vi "initialize.vi"(0 "mode":i32) -> ()   [LabVIEW 2015]
uses:
  phlib.dll
panel:
  out "Serial[8]":string="**********"
  in  "String2[8]":string="**********"
  out "Returncode PH_Initialize":i32
  out "Returncode PH_GetHardwareVersion":i32
  in  "String3[16]":string="*****************"
  in  "String4[8]":string="**********"
  out "DLL Version":string
  in  "String1[8]":string="**********"
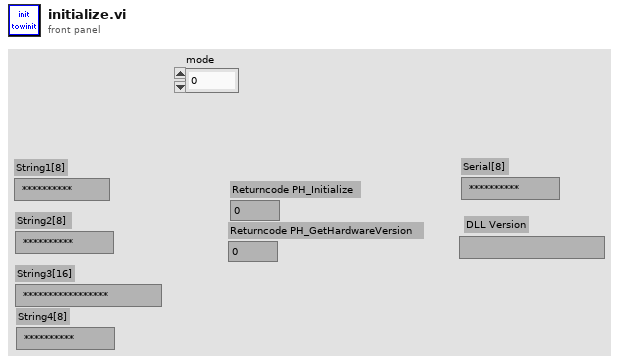
[diagram p1: front panel]
types:
  T1 = cluster{"initialized":bool, "devidx":i32, "Ch0 Level":i32, "Ch0 ZeroX":i32, "Ch1 Level":i32, "Ch1 ZeroX":i32, "sync rate":i32, "resolution":i32, "acq time":i32, "acq rate":i32, "# bins":u32, "Bin size":enum16{"1", "2", "4", "8", "16", "32", "64", "128"}, "min photons":u32, "truncate":u32}
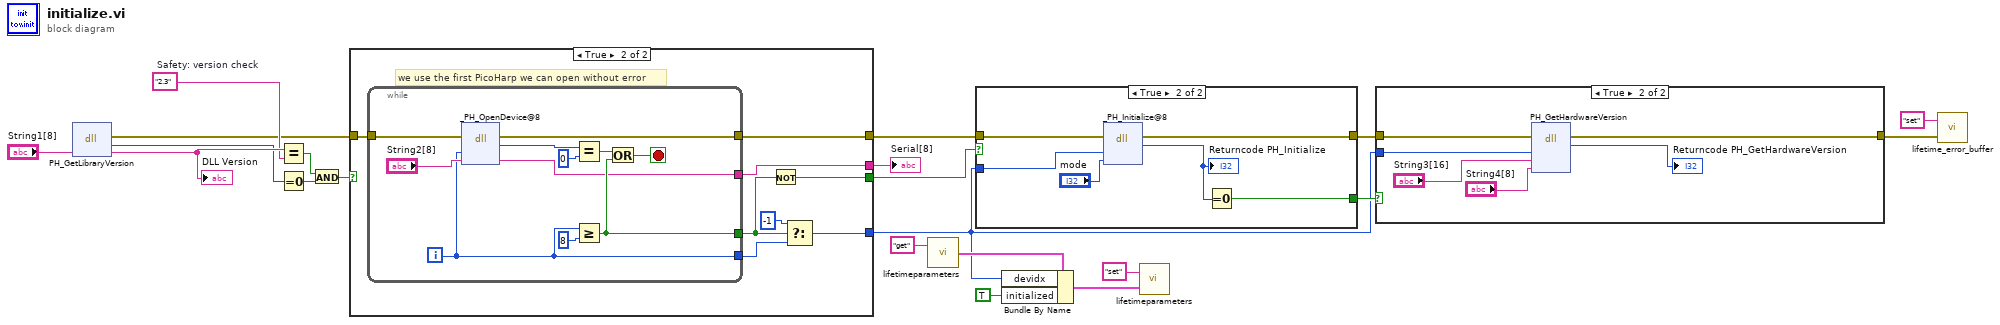
[diagram p0: block diagram]
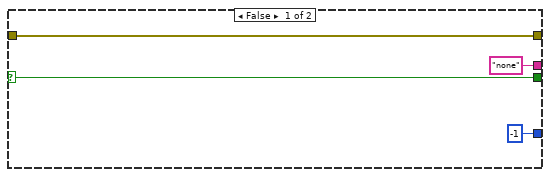
[diagram p2: hidden frame]
diagram:
  w19 = "2.3"  # Safety: version check
  n1 = dll-call lib="phlib.dll" fn="PH_GetLibraryVersion"("Version"="String1[8]") -> (error out=w5:errorcluster, w16:i32, "Version"=w20:string)  [unwired: 3 in, 1 out]
  "DLL Version" <- w20
  n2 = Equal?(x=w20, y=w19) -> (x = y?=w18:bool)
  n3 = Equal To 0?(x=w16) -> (x = 0?=w17:bool)
  n4 = And(x=w18, y=w17) -> (x .and. y?=w13:bool)
  n5 = case shown="True" w13 {
    selector: w13 -> [w25 _]
    tunnel: [w25 w29] -> w14
    tunnel: [-1 w32] -> w7
    tunnel: ["none" w28] -> w12
    tunnel: w5 -> [w22 w27]
    tunnel: [w22 w26] -> w4
    frame False {
    }
    frame True {
      # "we use the first PicoHarp we can open without error"
      n6 = while {
        tunnel: [w36] -> w28
        tunnel: [w40] -> w33
        tunnel: [w38] -> w30
        tunnel: w27 -> [w35]
        tunnel: [w34] -> w26
        i -> [w40]
        stop <- w37 stop-if-true
        n7 = dll-call lib="phlib.dll" fn="_PH_OpenDevice@8" label="PH_OpenDevice"(error in=w35, "devidx"=w40, "serial"="String2[8]") -> (error out=w34:errorcluster, w42:i32, "serial"=w36:string)  [unwired: 3 in, 1 out]
        n8 = Equal?(x=w42, y=0) -> (x = y?=w39:bool)
        n9 = Greater Or Equal?(x=w40, y=8) -> (x >= y?=w38:bool)
        n10 = Or(x=w39, y=w38) -> (x .or. y?=w37:bool)
      }
      n11 = Not(x=w30) -> (.not. x?=w29:bool)
      n12 = Select(t=-1, s=w30, f=w33) -> (s? t:f=w32:i32)
    }
  }
  "Serial[8]" <- w12
  n13 = call "lifetimeparameters.vi"("command"="get") -> ("Params out"=w8:T1)  [unwired: 1 in]
  n14 = case shown="True" w14 {
    selector: w14 -> [w46 _]
    tunnel: [w46 w51] -> w15
    tunnel: w7 -> [_ w50]
    tunnel: w4 -> [w45 w48]
    tunnel: [w45 w47] -> w3
    frame False {
    }
    frame True {
      n15 = dll-call lib="phlib.dll" fn="_PH_Initialize@8" label="PH_Initialize"(error in=w48, "devidx"=w50, "mode"="mode") -> (error out=w47:errorcluster, w52:i32)  [unwired: 4 in, 1 out]
      "Returncode PH_Initialize" <- w52
      n16 = Equal To 0?(x=w52) -> (x = 0?=w51:bool)
    }
  }
  n17 = Bundle By Name(cluster=w8, "devidx"=w7, "initialized"=TRUE) -> (w10:T1)
  n18 = call "lifetimeparameters.vi"("Params in"=w10, "command"="set") -> ()  [unwired: 1 out]
  n19 = case shown="True" w15 {
    tunnel: w7 -> [_ w58]
    tunnel: w3 -> [w53 w55]
    tunnel: [w53 w54] -> w2
    frame False {
    }
    frame True {
      n20 = dll-call lib="phlib.dll" fn="PH_GetHardwareVersion"(error in=w55, "devidx"=w58, "Model"="String3[16]", "Version"="String4[8]") -> (error out=w54:errorcluster, →"Returncode PH_GetHardwareVersion":i32)  [unwired: 5 in, 1 out]
    }
  }
  n21 = call "lifetime_error_buffer.vi"("error in"=w2, "command"="set") -> ()  [unwired: 1 out]
